vi "Bundle Script_Named (Un)Bundler Remove.vi"(8 "error in":errorcluster, 9 "Selected Item Indices":i32[](array[numeric]), 10 "Selected Items (tags)":string[](array[string]), 11 "Affected Items":T1) -> (0 "error out":errorcluster, 2 "Objects":refnum<vi>[](array[refnum]))   [LabVIEW 2023]
doc: "Takes teg list OR indices list. The latter so we can use this as a subVI easily."
uses:
  top/BundleMagic.ctl
panel:
  # "OR"
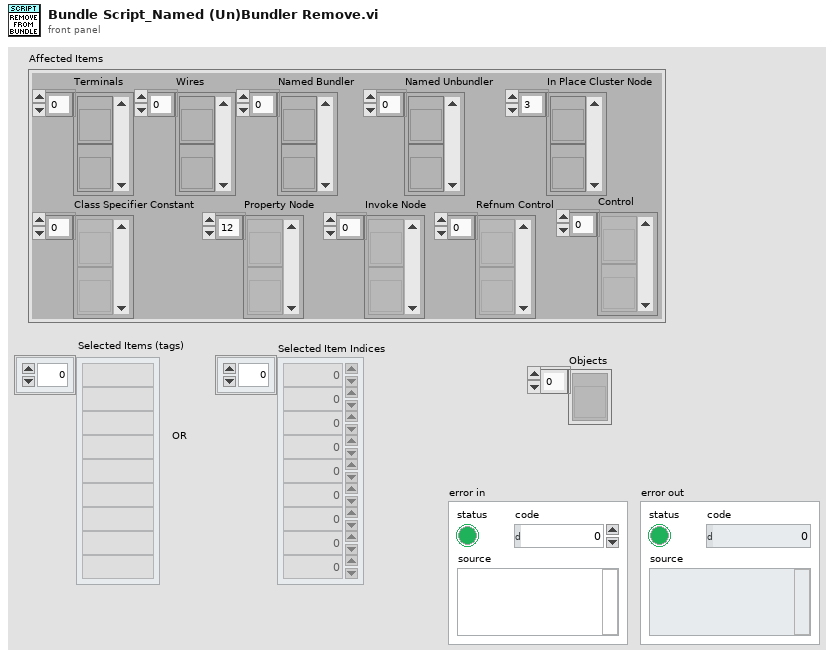
[diagram p1: front panel]
types:
  T1 = typedef "BundleMagic.ctl" = cluster{"Terminals":refnum<vi>[], "Wires":refnum<vi>[], "Named Bundler":refnum<vi>[], "Named Unbundler":refnum<vi>[], "In Place Cluster Node":refnum<vi>[], "Class Specifier Constant":refnum<vi>[], "Property Node":refnum<vi>[], "Invoke Node":refnum<vi>[], "Refnum Control":refnum<vi>[], "Control":refnum<vi>[]}
  T2 = enum16{"Named Bundler", "Named Unbundler", "In Place", "None"}
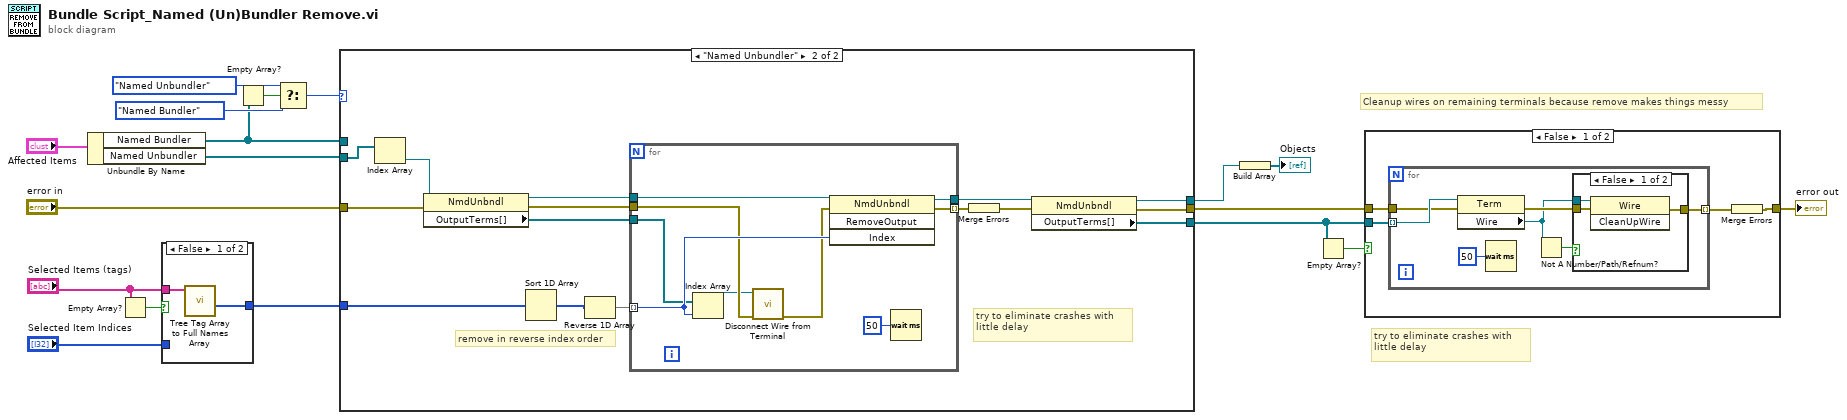
[diagram p0: block diagram]
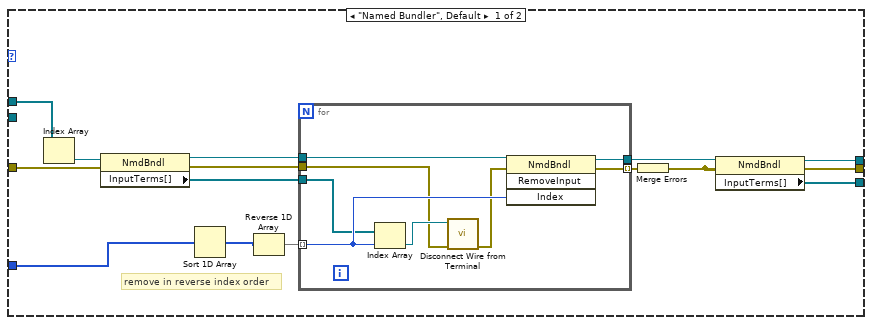
[diagram p5: hidden frame]
diagram:
  # "try to eliminate crashes with little delay"
  # "Cleanup wires on remaining terminals because remove makes things messy"
  n1 = Unbundle By Name("Affected Items") -> ("Named Bundler"=w12:refnum<vi>[], "Named Unbundler"=w11:refnum<vi>[])
  n2 = Empty Array?(array="Selected Items (tags)") -> (empty?=w3:bool)
  n3 = case shown="False" w3 {
    tunnel: "Selected Items (tags)" -> [w20 _]
    tunnel: [w19 w21] -> w9
    tunnel: "Selected Item Indices" -> [_ w21]
    frame False {
      n4 = call "Tree Tag Array to Full Names Array.vi"("Selected Items Tags"=w20) -> ("Selected Item Indices"=w19:u32[])  [unwired: 6 in, 4 out]
    }
    frame True {
    }
  }
  n5 = Empty Array?(array=w12) -> (empty?=w17:bool)
  n6 = Select(t=T2."Named Unbundler" ("Bundler Type"), s=w17, f=T2."Named Bundler" ("Bundler Type")) -> (s? t:f=w13:T2)
  n7 = case shown="\"Named Unbundler\"" w13 {
    tunnel: [w25 w46] -> w7
    tunnel: "error in" -> [w28 w52]
    tunnel: w12 -> [w27 _]
    tunnel: w11 -> [_ w51]
    tunnel: w9 -> [w26 w50]
    tunnel: [w22 w45] -> w8
    tunnel: [w23 w44] -> w5
    frame "Named Bundler", Default {
      # "remove in reverse index order"
      n8 = Index Array(array=w27) -> (element=w29:refnum<vi>)  [unwired: 1 in]
      n9 = property class="NmdBndl"(reference=w29, error in=w28) -> (reference out=w33:refnum<vi>, error out=w32:errorcluster, "InputTerms[]"=w31:refnum<vi>[])
      n10 = Sort 1D Array(array=w26) -> (sorted array=w35:u32[])
      n11 = Reverse 1D Array(array=w35) -> (reversed array=w34:u32[])
      n12 = for {
        tunnel: w34 -> [w43] mode=indexing
        tunnel: w33 -> [w42]
        tunnel: w32 -> [w37]
        tunnel: w31 -> [w41]
        tunnel: [w40] -> w30 mode=indexing
        tunnel: [w39] -> w24
        n13 = Index Array(array=w41, index=w43) -> (element=w38:refnum<vi>)
        n14 = call "Disconnect Wire from Terminal.vi"("error in"=w37, "Terminal in"=w38) -> ("error out"=w36:errorcluster)  [unwired: 5 in, 4 out]
        n15 = invoke class="NmdBndl" method="RemoveInput"(reference=w42, error in=w36, "Index"=w43) -> (reference out=w39:refnum<vi>, error out=w40:errorcluster)  [unwired: 1 in, 2 out]
      }
      n16 = Merge Errors(w30) -> (w25:errorcluster)
      n17 = property class="NmdBndl"(reference=w24, error in=w25) -> (reference out=w22:refnum<vi>, "InputTerms[]"=w23:refnum<vi>[])  [unwired: 1 out]
    }
    frame "Named Unbundler" {
      # "try to eliminate crashes with little delay"
      # "remove in reverse index order"
      n18 = Index Array(array=w51) -> (element=w53:refnum<vi>)  [unwired: 1 in]
      n19 = property class="NmdUnbndl"(reference=w53, error in=w52) -> (reference out=w56:refnum<vi>, error out=w55:errorcluster, "OutputTerms[]"=w49:refnum<vi>[])
      n20 = Sort 1D Array(array=w50) -> (sorted array=w58:u32[])
      n21 = Reverse 1D Array(array=w58) -> (reversed array=w57:u32[])
      n22 = for {
        tunnel: w57 -> [w67] mode=indexing
        tunnel: w56 -> [w66]
        tunnel: w55 -> [w62]
        tunnel: [w65] -> w54 mode=indexing
        tunnel: w49 -> [w64]
        tunnel: [w63] -> w48
        n23 = Index Array(array=w64, index=w67) -> (element=w60:refnum<vi>)
        n24 = call "Disconnect Wire from Terminal.vi"("error in"=w62, "Terminal in"=w60) -> ("error out"=w61:errorcluster)  [unwired: 5 in, 4 out]
        n25 = invoke class="NmdUnbndl" method="RemoveOutput"(reference=w66, error in=w61, "Index"=w67) -> (reference out=w63:refnum<vi>, error out=w65:errorcluster)  [unwired: 1 in, 2 out]
        n26 = Wait (ms)(milliseconds to wait=u32 50) -> ()  [unwired: 1 out]
      }
      n27 = Merge Errors(w54) -> (w47:errorcluster)
      n28 = property class="NmdUnbndl"(reference=w48, error in=w47) -> (reference out=w45:refnum<vi>, error out=w46:errorcluster, "OutputTerms[]"=w44:refnum<vi>[])
    }
  }
  n29 = Build Array(w8) -> (→"Objects":refnum<vi>[])
  n30 = Empty Array?(array=w5) -> (empty?=w4:bool)
  n31 = case shown="False" w4 {
    tunnel: w5 -> [w71 _]
    tunnel: w7 -> [w70 w83]
    tunnel: [w68 w83] -> w6
    frame False {
      n32 = for {
        tunnel: w71 -> [w77] mode=indexing
        tunnel: w70 -> [w76]
        tunnel: [w75] -> w69 mode=indexing
        n33 = property class="Term"(reference=w77, error in=w76) -> (error out=w78:errorcluster, "Wire"=w74:refnum<vi>)  [unwired: 1 out]
        n34 = Wait (ms)(milliseconds to wait=u32 50) -> ()  [unwired: 1 out]
        n35 = Not A Number/Path/Refnum?(number/path/refnum=w74) -> (NaN/Path/Refnum?=w73:bool)
        n36 = case shown="False" w73 {
          tunnel: w74 -> [w81 _]
          tunnel: w78 -> [w80 w82]
          tunnel: [w79 w82] -> w75
          frame False {
            n37 = invoke class="Wire" method="CleanUpWire"(reference=w81, error in=w80) -> (error out=w79:errorcluster)  [unwired: 1 in, 2 out]
          }
          frame True {
          }
        }
      }
      n38 = Merge Errors(w69) -> (w68:errorcluster)
    }
    frame True {
    }
  }
  "error out" <- w6
